vi "Query Instrument Status.vi"(8 "error in (no error)":errorcluster, 11 "VISA resource name":refnum<visa-resource-name>) -> (0 "error out":errorcluster, 2 "Instrument Status":T1, 3 "VISA resource name out":refnum<visa-resource-name>)   [LabVIEW 2014, in "Fluke 190 Series II.lvlib"]
doc: "Queries the contents of the Scopemeter's status register. The returned value reflects the present operational status of the testtool itself."
uses:
  Fluke 190 Series II.lvlib
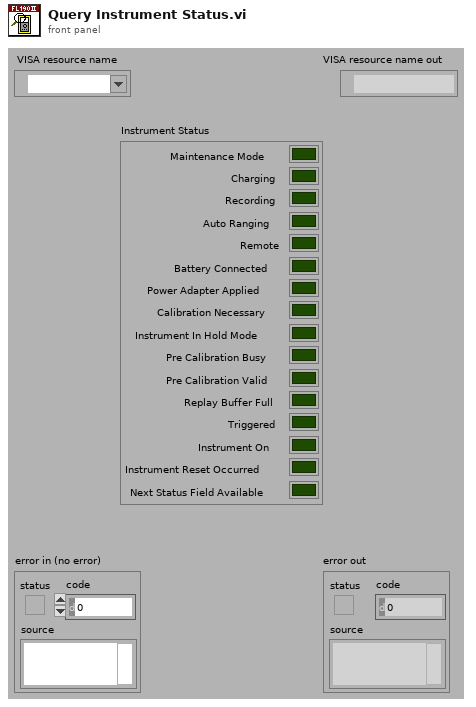
[diagram p1: front panel]
types:
  T1 = cluster{"Maintenance Mode":bool, "Charging":bool, "Recording":bool, "Auto Ranging":bool, "Remote":bool, "Battery Connected":bool, "Power Adapter Applied":bool, "Calibration Necessary":bool, "Instrument In Hold Mode":bool, "Pre Calibration Busy":bool, "Pre Calibration Valid":bool, "Replay Buffer Full":bool, "Triggered":bool, "Instrument On":bool, "Instrument Reset Occurred":bool, "Next Status Field Available":bool}
  T2 = cluster{bool, bool, bool, bool, bool, bool, bool, bool, bool, bool, bool, bool, bool, bool, bool, bool}
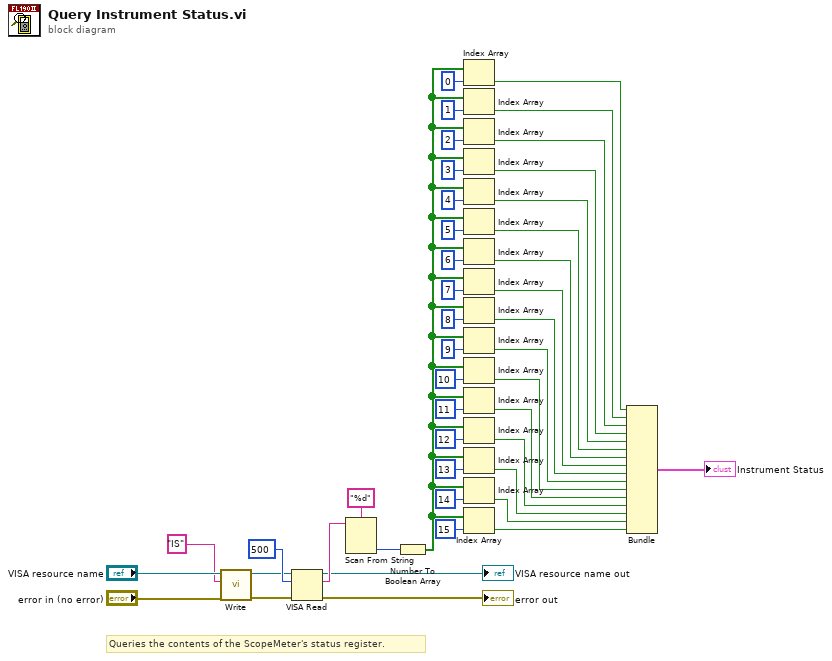
[diagram p0: block diagram]
diagram:
  # "Queries the contents of the ScopeMeter's status register."
  n1 = call "Write.vi"("error in (no error)"="error in (no error)", "Write Buffer"="IS", "VISA resource name"="VISA resource name") -> ("error out"=w39:errorcluster, "VISA resource name out"=w40:refnum<visa-resource-name>)  [unwired: 7 out]
  n2 = VISA Read(VISA resource name=w40, byte count=u32 500, error in (no error)=w39) -> (VISA resource name out=→"VISA resource name out":refnum<visa-resource-name>, read buffer=w44:string, error out=→"error out":errorcluster)  [unwired: 1 out]
  n3 = Scan From String(format string="%d", input string=w44) -> (output 1=w35:i32)  [unwired: 2 in, 4 out]
  n4 = Number To Boolean Array(number=w35) -> (Boolean array=w34:bool[])
  n5 = Index Array(array=w34, index=0) -> (element=w17:bool)
  n6 = Index Array(array=w34, index=1) -> (element=w15:bool)
  n7 = Index Array(array=w34, index=2) -> (element=w16:bool)
  n8 = Index Array(array=w34, index=3) -> (element=w1:bool)
  n9 = Index Array(array=w34, index=4) -> (element=w14:bool)
  n10 = Index Array(array=w34, index=5) -> (element=w13:bool)
  n11 = Index Array(array=w34, index=6) -> (element=w12:bool)
  n12 = Index Array(array=w34, index=7) -> (element=w11:bool)
  n13 = Index Array(array=w34, index=8) -> (element=w10:bool)
  n14 = Index Array(array=w34, index=9) -> (element=w9:bool)
  n15 = Index Array(array=w34, index=10) -> (element=w8:bool)
  n16 = Index Array(array=w34, index=11) -> (element=w7:bool)
  n17 = Index Array(array=w34, index=12) -> (element=w6:bool)
  n18 = Index Array(array=w34, index=13) -> (element=w5:bool)
  n19 = Index Array(array=w34, index=14) -> (element=w4:bool)
  n20 = Index Array(array=w34, index=15) -> (element=w3:bool)
  n21 = Bundle(w17, w15, w16, w1, w14, w13, w12, w11, w10, w9, w8, w7, w6, w5, w4, w3) -> (→"Instrument Status":T2)  [unwired: 1 out]
